vi "Load Config.vi"(6 "Constants":refnum<class "Sequence Constants.lvclass">, 8 "error in (no error)":refnum<class "MultiErrors.lvclass">, 10 "Config Element":refnum<class "Config Element.lvclass">, 11 "Stop Log Command Config in":refnum<class "Stop Log Command Config.lvclass">) -> (0 "error out":refnum<class "MultiErrors.lvclass">, 3 "Stop Log Command Config out":refnum<class "Stop Log Command Config.lvclass">)   [LabVIEW 2020, in "VolatusSeqConfig.lvlib" / "Stop Log Command Config.lvclass"]
uses:
  Stop Log Command Config.lvclass
  VolatusErrorUtilities/MultiErrors/MultiErrors.lvclass
  lv-cdm/CDM-Config/Config Element/Config Element.lvclass
  Stop Log Command Config.lvclass/Stop Log Command Config.ctl
  Sequence Constants/Sequence Constants.lvclass
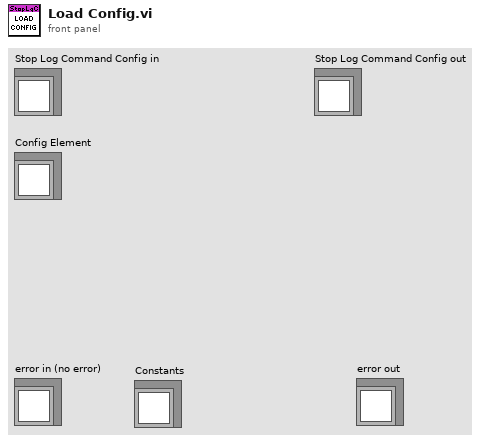
[diagram p1: front panel]
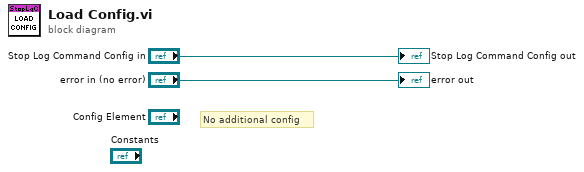
[diagram p0: block diagram]
diagram:
  # "No additional config"
  "error out" <- "error in (no error)"
  "Stop Log Command Config out" <- "Stop Log Command Config in"
